vi "laneleftright2.vi"() -> (2 "Coeff right":dbl[](array[numeric]), 3 "Coeff left":dbl[](array[numeric]))   [LabVIEW 2015]
uses:
  G_SEN.vi
  <vilib>/Analysis/1siggen.llb/Ramp Pattern by Delta.vi
  G_LCM.vi
  <vilib>/Analysis/polynomials.llb/1D Polynomial Evaluation (DBL).vi
  <vilib>/Analysis/NI_AALPro.lvlib
  <vilib>/Analysis/NI_AALBase.lvlib
panel:
  in  "poly":i32=5
  out "Coeff stop":dbl[](array[numeric])
  out "y_mobileye":dbl[](array[numeric])=[0.8601491478953653, 0.8717844136967624, 0.882947592858927, 0.8936326403234123, 0.9038337699485205, 0.9135454576426009, 0.9227624443554423, 0.9314797389261423, 0.9396926207859084, 0.9473966425143293, 0.9545876322477319, 0.9612616959383189, 0.9674152194628639, 0.9730448705798238, 0.9781476007338057, 0.9827206467064133, 0.9867615321125792, 0.9902680687415704, 0.993238357741943, 0.9956707906498045, 0.9975640502598242, 0.9989171113385246, 0.9997292411794617, 1.0, 0.9997292411794617, 0.9989171113385246, 0.9975640502598242, 0.9956707906498045, 0.993238357741943, 0.9902680687415704, 0.9867615321125792, 0.9827206467064133]
  in  "iter":i32=5
  out "Waveform Graph":dbl[](graph)
  out "w all":dbl[](array[numeric])
  out "c_tmp":dbl[](array[numeric])
  out "y seed":dbl[](array[numeric])
  out "XY Graph 4":cluster{"Y":dbl[], "Y":dbl[]}[](graph)=[{"Y"=array[3210 elements], "Y"=array[3210 elements]}, {"Y"=[-0.0, 0.001154394197769193, 0.004617650635850623, 0.010389990872226917, 0.018471784248973222, 0.02886354801042046, 0.041565947468740205, 0.056579796217107514, 0.0739060563904701, 0.0935458389742223, 0.11550040416098284, 0.13977116175580306, 0.16635967162997645, 0.19526764422393228, 0.2264969410994837, 0.26004957554195585, 0.2959277132125635, 0.3341336728515216, 0.374669927032528, 0.417539102969144, 0.4627439833735707, 0.5102875073687159, 0.560172771454063, 0.6124030305261954, 0.6669816989546717, 0.7239123517142048, 0.7831987255740245, 0.8448447203451934, 0.9088544001870815, 0.975231994973953, 1.0439819017227023, 1.1151086860829622, 1.1886170838907617, 1.2645120027869723, 1.342798523901962, 1.42348190360768, 1.5065675753387922, 1.592061151484188, 1.6799684253507792, 1.770295373200753, 1.8630481563645134, 1.9582331234307588, 2.0558568125157564, 2.1559259536137603, 2.258447471030621], "Y"=[0.0, 0.5, 1.0, 1.5, 2.0, 2.5, 3.0, 3.5, 4.0, 4.5, 5.0, 5.5, 6.0, 6.5, 7.0, 7.5, 8.0, 8.5, 9.0, 9.5, 10.0, 10.5, 11.0, 11.5, 12.0, 12.5, 13.0, 13.5, 14.0, 14.5, 15.0, 15.5, 16.0, 16.5, 17.0, 17.5, 18.0, 18.5, 19.0, 19.5, 20.0, 20.5, 21.0, 21.5, 22.0]}, {"Y"=[0.362252581831572], "Y"=[-0.8199241909738847]}, {"Y"=array[210 elements], "Y"=array[210 elements]}, {"Y"=[-0.925, -0.925, -0.925, -0.6775, -0.6775, -0.925, -0.925, -0.925, -0.925, -0.6775, -0.6775, -0.925, -0.925, -0.925, 0.9025, 0.9025, 0.9025, 0.6775, 0.6775, 0.9025, 0.9025, 0.9025, 0.9025, 0.6775, 0.6775, 0.9025, 0.9025, 0.9025, -0.925], "Y"=[-0.75, -0.224, 0.224, 0.224, -0.224, -0.224, 0.224, 2.415, 2.885, 2.885, 2.415, 2.415, 2.885, 3.5, 3.5, 2.885, 2.415, 2.415, 2.885, 2.885, 2.415, 0.224, -0.224, -0.224, 0.224, 0.224, -0.224, -0.75, -0.75]}, {"Y"=[0.171875, 0.15377271904051304, 0.1346290179491043, 0.11445423440635205, 0.09325870609283447, 0.07105277068912982, 0.04784676587581635, 0.02365102933347224, -0.0015241012573242174, -0.02766828821599482, -0.05477119386196136, -0.08282248051464558, -0.11181181049346922, -0.14172884611785413, -0.17256324970722198, -0.20430468358099463, -0.23694281005859374, -0.27046729145944115, -0.30486779010295867, -0.340133968308568, -0.3762554883956909, -0.41322201268374914, -0.4510232034921646, -0.4896487231403589], "Y"=[0.0, 0.5, 1.0, 1.5, 2.0, 2.5, 3.0, 3.5, 4.0, 4.5, 5.0, 5.5, 6.0, 6.5, 7.0, 7.5, 8.0, 8.5, 9.0, 9.5, 10.0, 10.5, 11.0, 11.5]}, {"Y"=[1.796875, 1.778772719040513, 1.7596290179491043, 1.739454234406352, 1.7182587060928345, 1.6960527706891297, 1.6728467658758164, 1.6486510293334722, 1.6234758987426758, 1.5973317117840051, 1.5702288061380387, 1.5421775194853544, 1.513188189506531, 1.483271153882146, 1.452436750292778, 1.4206953164190055, 1.3880571899414063, 1.354532708540559, 1.3201322098970414, 1.284866031691432, 1.248744511604309, 1.2117779873162509, 1.1739767965078354, 1.135351276859641, 1.0959117660522462, 1.0556686017662287, 1.014632121682167, 0.9728126634806396, 0.9302205648422242, 0.8868661634474992], "Y"=[0.0, 0.5, 1.0, 1.5, 2.0, 2.5, 3.0, 3.5, 4.0, 4.5, 5.0, 5.5, 6.0, 6.5, 7.0, 7.5, 8.0, 8.5, 9.0, 9.5, 10.0, 10.5, 11.0, 11.5, 12.0, 12.5, 13.0, 13.5, 14.0, 14.5]}, {"Y"=[-1.453125, -1.471227280959487, -1.4903709820508957, -1.510545765593648, -1.5317412939071655, -1.5539472293108703, -1.5771532341241836, -1.6013489706665278, -1.6265241012573242, -1.6526682882159949, -1.6797711938619613, -1.7078224805146456, -1.736811810493469, -1.766728846117854, -1.797563249707222, -1.8293046835809945, -1.8619428100585937, -1.895467291459441, -1.9298677901029586], "Y"=[0.0, 0.5, 1.0, 1.5, 2.0, 2.5, 3.0, 3.5, 4.0, 4.5, 5.0, 5.5, 6.0, 6.5, 7.0, 7.5, 8.0, 8.5, 9.0]}, {"Y"=[0.171875, 0.2568230007600336, 0.3384052130063493, 0.44574342526006827, 0.5205081969556753, 0.5917680690742042, 0.659409530134929, 0.7229937549325056, 0.7835496148685115, 0.8405449546633443, 0.9258576868463875], "Y"=[-20.239964538708662, -19.725637940364884, -19.211158961966362, -18.6998967366845, -18.19022720070031, -17.681887266143153, -17.17615515566314, -16.67683575591291, -16.176265245349786, -15.679082775270938, -15.183754484614711]}, {"Y"=[7.134647485270904], "Y"=[38.71960961082238]}, {"Y"=array[980 elements], "Y"=array[980 elements]}, {"Y"=[], "Y"=[]}]
  out "y all":dbl[](array[numeric])
  out "x all":dbl[](array[numeric])
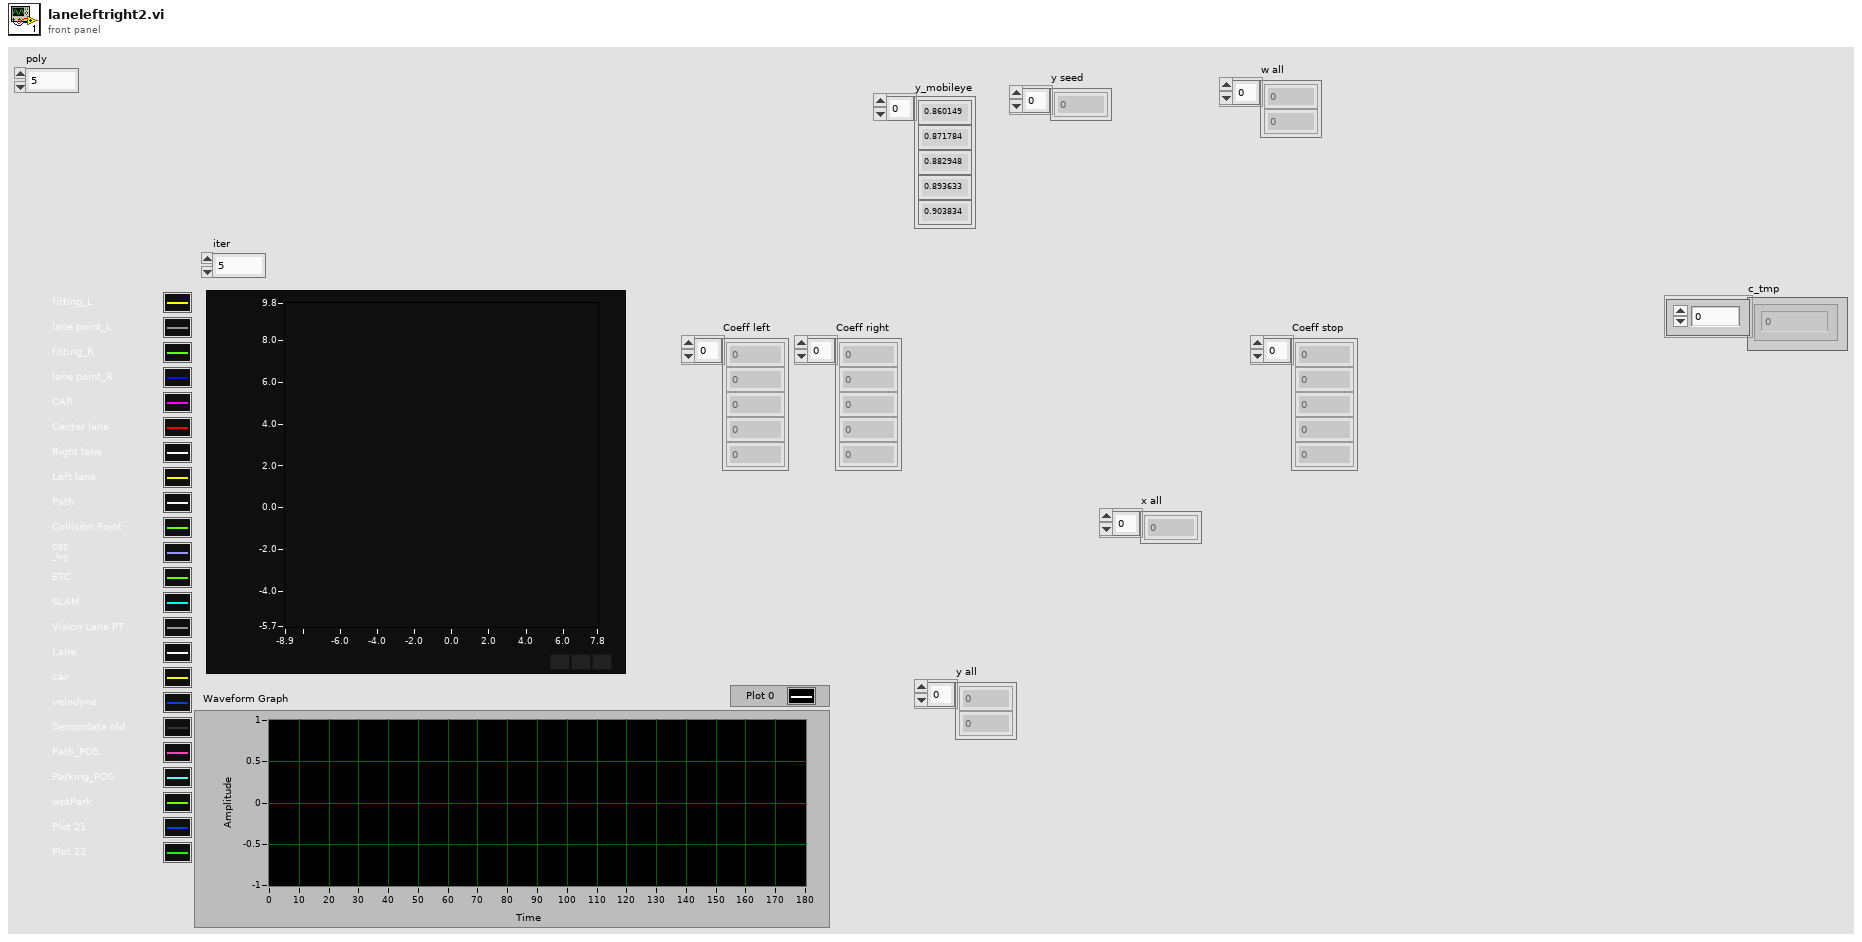
[diagram p1: front panel]
types:
  T1 = cluster{"hash":i64, "sys time":i64, "size":i64, "x":dbl[], "y":dbl[]}
  T2 = cluster{"delta":bool, "Rotational position":dbl, "Rotational position":dbl}[]
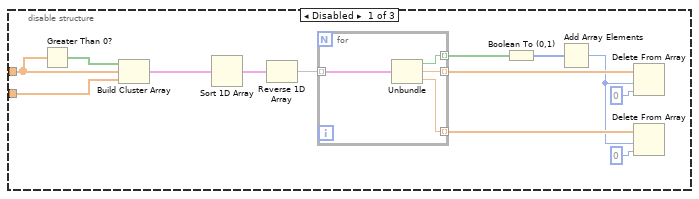
[diagram p4: hidden frame]
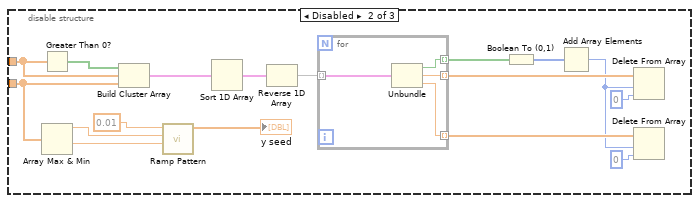
[diagram p5: hidden frame]
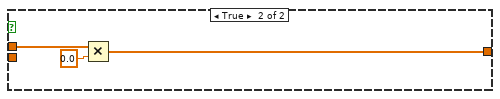
[diagram p6: hidden frame]
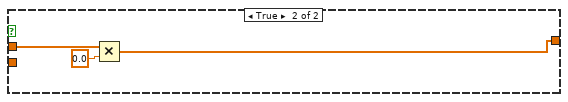
[diagram p7: hidden frame]
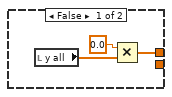
[diagram p8: hidden frame]
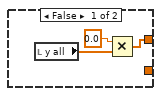
[diagram p9: hidden frame]
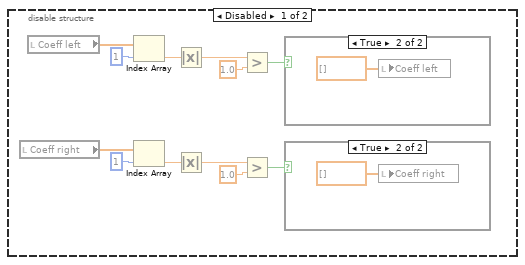
[diagram p11: hidden frame]
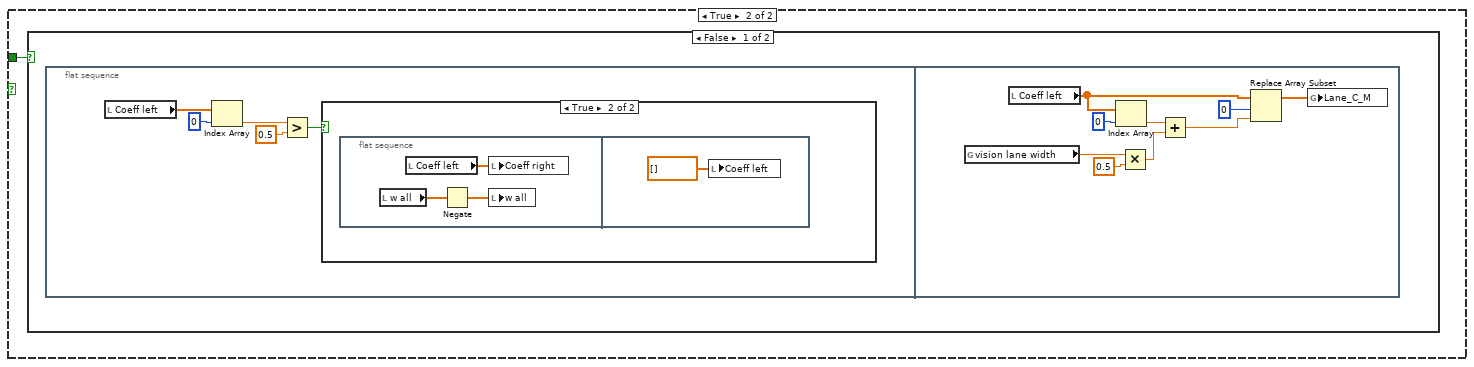
[diagram p15: hidden frame]
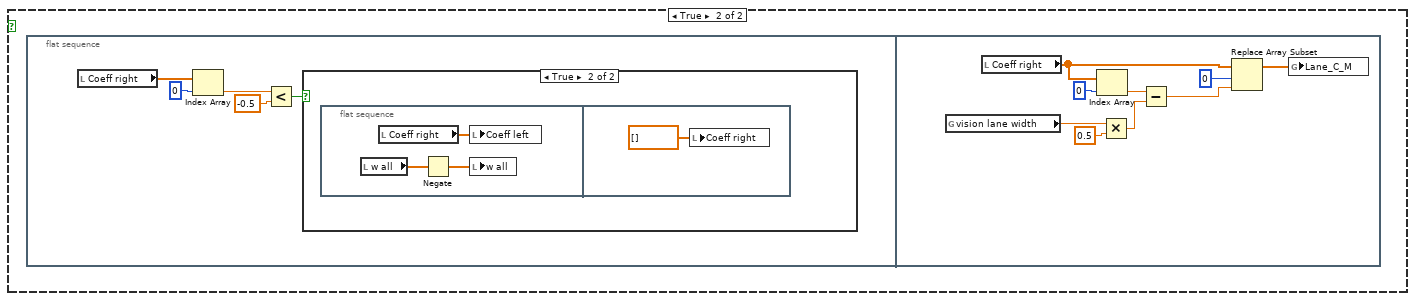
[diagram p17: hidden frame]
diagram:
  n1 = flat-sequence {
    frame #0 {
      n2 = First Call?() -> (First Call?: T/F=w1:bool)
      n3 = case shown="True" w1 {
        frame False {
        }
        frame True {
          w2 = dbl[][] [] ("Lane_R_V")
          n4 = disable-structure shown="Enabled" {
            frame Enabled {
              w8 = dbl[] [] ("Coeff left")
              n5 = local write "Coeff left"(w8) -> ()
              n6 = local write "Coeff right"(w8) -> ()
            }
            frame Disabled {
            }
          }
          n7 = global write "G_SEN.vi" "vision lane width"(3.5 ("vision lane width")) -> ()
          n8 = global write "G_SEN.vi" "Lane_L_V"(w2) -> ()
          n9 = global write "G_SEN.vi" "Lane_R_V"(w2) -> ()
          n10 = call-poly <vilib>:"Ramp Pattern.vi"("start"=-4.0, "end"=6.0, "delta"=0.1) -> ("Ramp Pattern"=→"y_mobileye":dbl[])  [unwired: 6 in, 2 out]
        }
      }
    }
    frame #1 {
      n11 = global read "G_LCM.vi" "VISION_LANE_PT"() -> (w26:T1)
      n12 = Unbundle By Name(w26) -> ("x"=w15:dbl[], "y"=w14:dbl[])
      n13 = In Range and Coerce(upper limit=6.0 ("delta"), x=w14, lower limit=-4.0) -> (In Range?=w17:bool[])  [unwired: 1 out]
      n14 = Build Cluster Array(w17, w15, w14) -> (w19:T2)
      n15 = Sort 1D Array(array=w19) -> (sorted array=w18:T2)
      n16 = Reverse 1D Array(array=w18) -> (reversed array=w24:T2)
      n17 = for {
        tunnel: w24 -> [w30] mode=indexing
        tunnel: [w29] -> w22 mode=indexing
        tunnel: [w28] -> w21 mode=indexing
        tunnel: [w27] -> w13 mode=indexing
        n18 = Unbundle(w30) -> ("delta"=w27:bool, "Rotational position"=w29:dbl, "Rotational position"=w28:dbl)
      }
      n19 = Boolean To (0,1)(Boolean=w13) -> (0, 1=w23:i16[])
      n20 = Add Array Elements(numeric array=w23) -> (sum=w12:i16)
      n21 = Delete From Array(array=w22, length=w12, index=0) -> (deleted portion=→"x all":dbl[])  [unwired: 1 out]
      n22 = Delete From Array(array=w21, length=w12, index=0) -> (deleted portion=→"y all":dbl[])  [unwired: 1 out]
    }
    frame #2 {
      n23 = local read "x all"() -> (w33:dbl[])
      n24 = local read "y all"() -> (w32:dbl[])
      n25 = disable-structure shown="Enabled" {
        disable-tunnel: w33 -> [w35 w56 w92]
        disable-tunnel: w32 -> [w46 w55 w97]
        disable-tunnel: [_ _ w72] -> w31
        frame Disabled {
          n26 = Greater Than 0?(x=w35) -> (x > 0?=w34:bool[])
          n27 = Build Cluster Array(w34, w35, w46) -> (w45:cluster{bool, dbl, dbl}[])
          n28 = Sort 1D Array(array=w45) -> (sorted array=w44:cluster{bool, dbl, dbl}[])
          n29 = Reverse 1D Array(array=w44) -> (reversed array=w43:cluster{bool, dbl, dbl}[])
          n30 = for {
            tunnel: w43 -> [w50] mode=indexing
            tunnel: [w49] -> w40 mode=indexing
            tunnel: [w48] -> w39 mode=indexing
            tunnel: [w47] -> w42 mode=indexing
            n31 = Unbundle(w50) -> (w47:bool, w49:dbl, w48:dbl)
          }
          n32 = Boolean To (0,1)(Boolean=w42) -> (0, 1=w41:i16[])
          n33 = Add Array Elements(numeric array=w41) -> (sum=w38:i16)
          n34 = Delete From Array(array=w40, length=w38, index=0) -> ()  [unwired: 2 out]
          n35 = Delete From Array(array=w39, length=w38, index=0) -> ()  [unwired: 2 out]
        }
        frame Disabled {
          n36 = Greater Than 0?(x=w56) -> (x > 0?=w57:bool[])
          n37 = Array Max & Min(array=w55) -> (max value=w54:dbl, min value=w53:dbl)  [unwired: 2 out]
          n38 = Build Cluster Array(w57, w56, w55) -> (w67:cluster{bool, dbl, dbl}[])
          n39 = call-poly <vilib>:"Ramp Pattern.vi"("start"=w53, "end"=w54, "delta"=0.01) -> ("Ramp Pattern"=→"y seed":dbl[])  [unwired: 6 in, 2 out]
          n40 = Sort 1D Array(array=w67) -> (sorted array=w66:cluster{bool, dbl, dbl}[])
          n41 = Reverse 1D Array(array=w66) -> (reversed array=w65:cluster{bool, dbl, dbl}[])
          n42 = for {
            tunnel: w65 -> [w71] mode=indexing
            tunnel: [w70] -> w62 mode=indexing
            tunnel: [w69] -> w61 mode=indexing
            tunnel: [w68] -> w64 mode=indexing
            n43 = Unbundle(w71) -> (w68:bool, w70:dbl, w69:dbl)
          }
          n44 = Boolean To (0,1)(Boolean=w64) -> (0, 1=w63:i16[])
          n45 = Add Array Elements(numeric array=w63) -> (sum=w60:i16)
          n46 = Delete From Array(array=w62, length=w60, index=0) -> ()  [unwired: 2 out]
          n47 = Delete From Array(array=w61, length=w60, index=0) -> ()  [unwired: 2 out]
        }
        frame Enabled {
          n48 = Subtract(x=w92, y=6.0) -> (x-y=w105:dbl[])
          n49 = Subtract(x=w97, y=0.0) -> (x-y=w95:dbl[])
          n50 = Subtract(x=w92, y=-6.0) -> (x-y=w103:dbl[])
          n51 = local read "Coeff left"() -> (w76:dbl[])
          n52 = Square(x=w103) -> (x^2=w104:dbl[])
          n53 = Square(x=w105) -> (x^2=w94:dbl[])
          n54 = Square(x=w95) -> (x^2=w93:dbl[])
          n55 = local read "Coeff right"() -> (w77:dbl[])
          n56 = Add(x=w104, y=w93) -> (x+y=w86:dbl[])
          n57 = Add(x=w93, y=w94) -> (x+y=w91:dbl[])
          n58 = Empty Array?(array=w76) -> (empty?=w75:bool)
          n59 = local read "y all"() -> (w79:dbl[])
          n60 = Empty Array?(array=w77) -> (empty?=w74:bool)
          n61 = In Range and Coerce(upper limit=36.0, x=w86, lower limit=4.0) -> (In Range?=w84:bool[])  [unwired: 1 out]
          n62 = In Range and Coerce(upper limit=36.0, x=w91, lower limit=4.0) -> (In Range?=w85:bool[])  [unwired: 1 out]
          n63 = local read "y all"() -> (w73:dbl[])
          n64 = case shown="False" w75 {
            tunnel: w79 -> [w126 w134]
            tunnel: w76 -> [w123 _]
            tunnel: [w121 w133] -> w78
            frame False {
              n65 = call-poly <vilib>:"Polynomial Evaluation.vi"("P(x)"=w123, "A"=w126) -> ("P(A)"=w125:dbl[])  [unwired: 1 out]
              n66 = local read "x all"() -> (w124:dbl[])
              n67 = Subtract(x=w125, y=w124) -> (x-y=w130:dbl[])
              n68 = Absolute Value(x=w130) -> (abs(x)=w129:dbl[])
              n69 = Negate(x=w129) -> (-x=w128:dbl[])
              n70 = Add(x=w128, y=1.0) -> (x+y=w132:dbl[])
              n71 = Max & Min(x=0.0, y=w132) -> (max(x,y)=w122:dbl[])  [unwired: 1 out]
              n72 = Negate(x=w122) -> (-x=w121:dbl[])
            }
            frame True {
              n73 = Multiply(x=w134, y=0.0) -> (x*y=w133:dbl[])
            }
          }
          n74 = case shown="False" w74 {
            tunnel: [w115 w118] -> w81
            tunnel: w77 -> [w114 _]
            tunnel: w73 -> [w107 w119]
            frame False {
              n75 = call-poly <vilib>:"Polynomial Evaluation.vi"("P(x)"=w114, "A"=w107) -> ("P(A)"=w112:dbl[])  [unwired: 1 out]
              n76 = local read "x all"() -> (w113:dbl[])
              n77 = Subtract(x=w112, y=w113) -> (x-y=w108:dbl[])
              n78 = Absolute Value(x=w108) -> (abs(x)=w109:dbl[])
              n79 = Negate(x=w109) -> (-x=w110:dbl[])
              n80 = Add(x=w110, y=1.0) -> (x+y=w116:dbl[])
              n81 = Max & Min(x=0.0, y=w116) -> (max(x,y)=w115:dbl[])  [unwired: 1 out]
            }
            frame True {
              n82 = Multiply(x=w119, y=0.0) -> (x*y=w118:dbl[])
            }
          }
          n83 = Boolean To (0,1)(Boolean=w84) -> (0, 1=w83:i16[])
          n84 = Boolean To (0,1)(Boolean=w85) -> (0, 1=w82:i16[])
          n85 = Multiply(x=i16 -1, y=w83) -> (x*y=w100:i16[])
          n86 = Add(x=w100, y=w82) -> (x+y=w98:i16[])
          n87 = Multiply(x=w98, y=1.0 ("element")) -> (x*y=w80:dbl[])
          n88 = Compound Arithmetic op=ADD(w80, w81, w78) -> (w72:dbl[])
        }
      }
      "w all" <- w31
    }
    frame #3 {
      n89 = for {
        N: "iter" -> [_]
        tunnel: "poly" -> [w139]
        n90 = flat-sequence {
          tunnel: [w153] -> w145
          tunnel: w139 -> [w146]
          tunnel: [w146] -> w138
          tunnel: [w184] -> w144
          tunnel: w145 -> [w184]
          tunnel: [w181] -> w142
          tunnel: w138 -> [w174]
          tunnel: w144 -> [w246]
          tunnel: [w246] -> w143
          tunnel: w142 -> [w245]
          tunnel: [w245] -> w141
          tunnel: [w216] -> w140
          tunnel: w143 -> [w254]
          tunnel: w141 -> [w253]
          tunnel: w140 -> [w252]
          frame #0 {
            n91 = local read "w all"() -> (w155:dbl[])
            n92 = Greater?(x=w155, y=0.99) -> (0:w147:bool[])
            n93 = Boolean To (0,1)(Boolean=w147) -> (0, 1=w148:i16[])
            n94 = Add Array Elements(numeric array=w148) -> (sum=w151:i16)
            n95 = Greater?(x=w151, y=i16 50) -> (0:w149:bool)
            n96 = case shown="True" w149 {
              tunnel: [w157 w164] -> w153
              tunnel: [_ w163] -> w152
              tunnel: w148 -> [_ w160]
              tunnel: w146 -> [_ w159]
              frame False {
                n97 = local read "y all"() -> (w158:dbl[])
                n98 = Multiply(x=0.0, y=w158) -> (x*y=w157:dbl[])
              }
              frame True {
                n99 = local read "x all"() -> (w161:dbl[])
                n100 = local read "y all"() -> (w162:dbl[])
                n101 = call <vilib>:"General Polynomial Fit Coefficients.vi"("Y"=w161, "polynomial order"=w159, "X"=w162, "Weight"=w160) -> ("Polynomial Coefficients"=w163:dbl[])  [unwired: 10 in, 1 out]
                n102 = local read "y all"() -> (w173:dbl[])
                n103 = call-poly <vilib>:"Polynomial Evaluation.vi"("P(x)"=w163, "A"=w173) -> ("P(A)"=w172:dbl[])  [unwired: 1 out]
                n104 = local read "x all"() -> (w171:dbl[])
                n105 = Subtract(x=w172, y=w171) -> (x-y=w170:dbl[])
                n106 = Absolute Value(x=w170) -> (abs(x)=w169:dbl[])
                n107 = Negate(x=w169) -> (-x=w168:dbl[])
                n108 = Add(x=w168, y=1.0) -> (x+y=w165:dbl[])
                n109 = Max & Min(x=0.0, y=w165) -> (max(x,y)=w164:dbl[])  [unwired: 1 out]
              }
            }
            "Coeff right" <- w152
          }
          frame #1 {
            n110 = local read "w all"() -> (w182:dbl[])
            n111 = Less?(x=w182, y=-0.99) -> (x < y?=w177:bool[])
            n112 = Boolean To (0,1)(Boolean=w177) -> (0, 1=w175:i16[])
            n113 = Add Array Elements(numeric array=w175) -> (sum=w178:i16)
            n114 = Greater?(x=w178, y=i16 50) -> (0:w176:bool)
            n115 = case shown="True" w176 {
              tunnel: [w185 w193] -> w181
              tunnel: [_ w192] -> w180
              tunnel: w175 -> [_ w189]
              tunnel: w174 -> [_ w188]
              frame False {
                n116 = local read "y all"() -> (w186:dbl[])
                n117 = Multiply(x=0.0, y=w186) -> (x*y=w185:dbl[])
              }
              frame True {
                n118 = local read "x all"() -> (w190:dbl[])
                n119 = local read "y all"() -> (w191:dbl[])
                n120 = call <vilib>:"General Polynomial Fit Coefficients.vi"("Y"=w190, "polynomial order"=w188, "X"=w191, "Weight"=w189) -> ("Polynomial Coefficients"=w192:dbl[])  [unwired: 10 in, 1 out]
                n121 = local read "y all"() -> (w197:dbl[])
                n122 = call-poly <vilib>:"Polynomial Evaluation.vi"("P(x)"=w192, "A"=w197) -> ("P(A)"=w198:dbl[])  [unwired: 1 out]
                n123 = local read "x all"() -> (w199:dbl[])
                n124 = Subtract(x=w198, y=w199) -> (x-y=w200:dbl[])
                n125 = Absolute Value(x=w200) -> (abs(x)=w201:dbl[])
                n126 = Negate(x=w201) -> (-x=w195:dbl[])
                n127 = Add(x=w195, y=1.0) -> (x+y=w202:dbl[])
                n128 = Max & Min(x=0.0, y=w202) -> (max(x,y)=w196:dbl[])  [unwired: 1 out]
                n129 = Negate(x=w196) -> (-x=w193:dbl[])
              }
            }
            "Coeff left" <- w180
          }
          frame #2 {
            n130 = local read "w all"() -> (w224:dbl[])
            n131 = local read "y all"() -> (w228:dbl[])
            n132 = Absolute Value(x=w224) -> (abs(x)=w223:dbl[])
            n133 = Greater?(x=w228, y=2.0) -> (0:w226:bool[])
            n134 = Less?(x=w223, y=0.25) -> (x < y?=w222:bool[])
            n135 = And(x=w226, y=w222) -> (x .and. y?=w225:bool[])
            n136 = Boolean To (0,1)(Boolean=w225) -> (0, 1=w244:i16[])
            n137 = local read "y all"() -> (w238:dbl[])
            n138 = local read "x all"() -> (w237:dbl[])
            n139 = call <vilib>:"General Polynomial Fit Coefficients.vi"("Y"=w238, "polynomial order"=1, "X"=w237, "Weight"=w244) -> ("Polynomial Coefficients"=w209:dbl[])  [unwired: 10 in, 1 out]
            n140 = local read "x all"() -> (w242:dbl[])
            n141 = Equal To 0?(x=w209) -> (x = 0?=w208:bool[])
            n142 = Index Array(array=w209, index=1) -> (element=w219:dbl)
            n143 = And Array Elements(Boolean array=w208) -> (logical AND=w205:bool)
            n144 = call-poly <vilib>:"Polynomial Evaluation.vi"("P(x)"=w209, "A"=w242) -> ("P(A)"=w241:dbl[])  [unwired: 1 out]
            n145 = In Range and Coerce(upper limit=0.5, x=w219, lower limit=-0.5) -> (In Range?=w207:bool)  [unwired: 1 out]
            n146 = local read "y all"() -> (w240:dbl[])
            n147 = Not(x=w205) -> (.not. x?=w204:bool)
            n148 = Subtract(x=w241, y=w240) -> (x-y=w239:dbl[])
            n149 = disable-structure shown="Enabled" {
              disable-tunnel: w207 -> [w249 _]
              disable-tunnel: [w248 _] -> w206
              disable-tunnel: w204 -> [w247 _]
              frame Enabled {
                n150 = And(x=w247, y=w249) -> (x .and. y?=w248:bool)
              }
              frame Disabled {
              }
            }
            n151 = Absolute Value(x=w239) -> (abs(x)=w236:dbl[])
            n152 = Greater?(x=w236, y=0.25 ("Numeric 2")) -> (0:w234:bool[])
            n153 = Not(x=w234) -> (.not. x?=w233:bool[])
            n154 = Boolean To (0,1)(Boolean=w234) -> (0, 1=w229:i16[])
            n155 = Boolean To (0,1)(Boolean=w233) -> (0, 1=w232:i16[])
            n156 = Select(t=w209, s=w206, f=dbl[] []) -> (s? t:f=→"Coeff stop":dbl[])
            n157 = Multiply(x=w232, y=0.5) -> (x*y=w230:dbl[])
            n158 = Add(x=w229, y=w230) -> (x+y=w215:dbl[])
            n159 = Multiply(x=w215, y=0.0) -> (x*y=w213:dbl[])
            n160 = Increment(x=w213) -> (x+1=w212:dbl[])
            n161 = Select(t=w215, s=w206, f=w212) -> (s? t:f=w216:dbl[])
          }
          frame #3 {
            n162 = local read "w all"() -> (w258:dbl[])
            n163 = Compound Arithmetic op=ADD(w258, w254, w253) -> (w251:dbl[])
            n164 = Multiply(x=w252, y=w251) -> (x*y=w250:dbl[])
            n165 = In Range and Coerce(upper limit=1.0, x=w250, lower limit=-1.0) -> (coerced(x)=w255:dbl[])  [unwired: 1 out]
            n166 = local write "w all"(w255) -> ()
          }
        }
      }
    }
    frame #4 {
      n167 = disable-structure shown="Enabled" {
        frame Disabled {
          n168 = local read "Coeff right"() -> (w261:dbl[])
          n169 = local read "Coeff left"() -> (w268:dbl[])
          n170 = Index Array(array=w268, index=1) -> (element=w267:dbl)
          n171 = Index Array(array=w261, index=1) -> (element=w262:dbl)
          n172 = Absolute Value(x=w267) -> (abs(x)=w270:dbl)
          n173 = Absolute Value(x=w262) -> (abs(x)=w259:dbl)
          n174 = Greater?(x=w270, y=1.0) -> (0:w265:bool)
          n175 = Greater?(x=w259, y=1.0) -> (0:w264:bool)
          n176 = case shown="True" w265 {
            frame False {
            }
            frame True {
              n177 = local write "Coeff left"(dbl[] [] ("Coeff left")) -> ()
            }
          }
          n178 = case shown="True" w264 {
            frame False {
            }
            frame True {
              n179 = local write "Coeff right"(dbl[] [] ("Coeff left")) -> ()
            }
          }
        }
        frame Enabled {
          w289 = 4 ("Numeric 2")
          n180 = local read "Coeff right"() -> (w291:dbl[])
          n181 = local read "Coeff left"() -> (w293:dbl[])
          n182 = Array Subset(array=w293, index=0, length=w289) -> (w274:dbl[])
          n183 = Array Subset(array=w291, index=0, length=w289) -> (w283:dbl[])
          n184 = Index Array(array=w274, index=1) -> (element=w276:dbl)
          n185 = Index Array(array=w283, index=1) -> (element=w287:dbl)
          n186 = Absolute Value(x=w276) -> (abs(x)=w277:dbl)
          n187 = Absolute Value(x=w287) -> (abs(x)=w286:dbl)
          n188 = Less?(x=w277, y=1.0) -> (x < y?=w279:bool)
          n189 = Less?(x=w286, y=1.0) -> (x < y?=w284:bool)
          n190 = Select(t=w274, s=w279, f=dbl[] []) -> (s? t:f=w273:dbl[])
          n191 = Select(t=w283, s=w284, f=dbl[] []) -> (s? t:f=w282:dbl[])
          n192 = local write "Coeff left"(w273) -> ()
          n193 = local write "Coeff right"(w282) -> ()
        }
      }
    }
    frame #5 {
      n194 = disable-structure shown="Enabled" {
        frame Enabled {
          n195 = local read "Coeff right"() -> (w297:dbl[])
          n196 = local read "Coeff left"() -> (w298:dbl[])
          n197 = Empty Array?(array=w298) -> (empty?=w294:bool)
          n198 = Empty Array?(array=w297) -> (empty?=w296:bool)
          n199 = Exclusive Or(1:w296, 2:w294) -> (0:w295:bool)
          n200 = case shown="False" w295 {
            tunnel: w294 -> [_ w320]
            frame False {
              n201 = flat-sequence {
                frame #0 {
                  n202 = local read "Coeff right"() -> (w302:dbl[])
                  n203 = local read "Coeff left"() -> (w303:dbl[])
                  n204 = Index Array(array=w303) -> (element=w301:dbl)  [unwired: 1 in]
                  n205 = Index Array(array=w302) -> (element=w300:dbl)  [unwired: 1 in]
                  n206 = Greater?(x=w301, y=w300) -> (0:w299:bool)
                  n207 = case shown="True" w299 {
                    frame False {
                    }
                    frame True {
                      n208 = flat-sequence {
                        frame #0 {
                          n209 = local read "Coeff right"() -> (→"c_tmp":dbl[])
                        }
                        frame #1 {
                          n210 = local read "w all"() -> (w306:dbl[])
                          n211 = local read "Coeff left"() -> (w307:dbl[])
                          n212 = Negate(x=w306) -> (-x=w305:dbl[])
                          n213 = local write "Coeff right"(w307) -> ()
                          n214 = local write "w all"(w305) -> ()
                        }
                        frame #2 {
                          n215 = local read "c_tmp"() -> (w308:dbl[])
                          n216 = local write "Coeff left"(w308) -> ()
                        }
                      }
                    }
                  }
                }
                frame #1 {
                  n217 = local read "Coeff right"() -> (w314:dbl[])
                  n218 = local read "Coeff left"() -> (w317:dbl[])
                  n219 = local read "Coeff left"() -> (w313:dbl[])
                  n220 = Subtract(x=w314, y=w317) -> (x-y=w316:dbl[])
                  n221 = Add(x=w313, y=w314) -> (x+y=w319:dbl[])
                  n222 = Index Array(array=w316, index=0) -> (element=w311:dbl)
                  n223 = Multiply(x=w319, y=0.5) -> (x*y=w312:dbl[])
                  n224 = global write "G_SEN.vi" "Lane_C_M"(w312) -> ()
                  n225 = Max & Min(x=w311, y=3.2) -> (max(x,y)=w310:dbl)  [unwired: 1 out]
                  n226 = global write "G_SEN.vi" "vision lane width"(w310) -> ()
                }
              }
            }
            frame True {
              n227 = case shown="False" w320 {
                frame False {
                  n228 = flat-sequence {
                    frame #0 {
                      n229 = local read "Coeff left"() -> (w325:dbl[])
                      n230 = Index Array(array=w325, index=0) -> (element=w323:dbl)
                      n231 = Greater?(x=w323, y=0.5) -> (0:w321:bool)
                      n232 = case shown="True" w321 {
                        frame False {
                        }
                        frame True {
                          n233 = flat-sequence {
                            frame #0 {
                              n234 = local read "w all"() -> (w327:dbl[])
                              n235 = local read "Coeff left"() -> (w328:dbl[])
                              n236 = Negate(x=w327) -> (-x=w326:dbl[])
                              n237 = local write "Coeff right"(w328) -> ()
                              n238 = local write "w all"(w326) -> ()
                            }
                            frame #1 {
                              n239 = local write "Coeff left"(dbl[] []) -> ()
                            }
                          }
                        }
                      }
                    }
                    frame #1 {
                      n240 = global read "G_SEN.vi" "vision lane width"() -> (w338:dbl)
                      n241 = local read "Coeff left"() -> (w336:dbl[])
                      n242 = Index Array(array=w336, index=0) -> (element=w334:dbl)
                      n243 = Multiply(x=w338, y=0.5) -> (x*y=w333:dbl)
                      n244 = Add(x=w334, y=w333) -> (x+y=w332:dbl)
                      n245 = Replace Array Subset(array=w336, new element=w332, index=0) -> (w330:dbl[])
                      n246 = global write "G_SEN.vi" "Lane_C_M"(w330) -> ()
                    }
                  }
                }
                frame True {
                  n247 = flat-sequence {
                    frame #0 {
                      n248 = local read "Coeff right"() -> (w343:dbl[])
                      n249 = Index Array(array=w343, index=0) -> (element=w341:dbl)
                      n250 = Less?(x=w341, y=-0.5) -> (x < y?=w339:bool)
                      n251 = case shown="True" w339 {
                        frame False {
                        }
                        frame True {
                          n252 = flat-sequence {
                            frame #0 {
                              n253 = local read "w all"() -> (w345:dbl[])
                              n254 = local read "Coeff right"() -> (w346:dbl[])
                              n255 = Negate(x=w345) -> (-x=w344:dbl[])
                              n256 = local write "Coeff left"(w346) -> ()
                              n257 = local write "w all"(w344) -> ()
                            }
                            frame #1 {
                              n258 = local write "Coeff right"(dbl[] []) -> ()
                            }
                          }
                        }
                      }
                    }
                    frame #1 {
                      n259 = global read "G_SEN.vi" "vision lane width"() -> (w356:dbl)
                      n260 = local read "Coeff right"() -> (w354:dbl[])
                      n261 = Index Array(array=w354, index=0) -> (element=w352:dbl)
                      n262 = Multiply(x=w356, y=0.5) -> (x*y=w351:dbl)
                      n263 = Subtract(x=w352, y=w351) -> (x-y=w350:dbl)
                      n264 = Replace Array Subset(array=w354, new element=w350, index=0) -> (w348:dbl[])
                      n265 = global write "G_SEN.vi" "Lane_C_M"(w348) -> ()
                    }
                  }
                }
              }
            }
          }
        }
        frame Disabled {
        }
      }
    }
    frame #6 {
      n266 = local read "w all"() -> (→"Waveform Graph":dbl[])
      n267 = disable-structure shown="Enabled" {
        frame Enabled {
          n268 = local read "Coeff right"() -> (w358:dbl[])
          n269 = local read "Coeff left"() -> (w359:dbl[])
          n270 = global write "G_SEN.vi" "Lane_R_M"(w358) -> ()
          n271 = global write "G_SEN.vi" "Lane_L_M"(w359) -> ()
        }
        frame Disabled {
        }
      }
    }
    frame #7 {
      n272 = local read "w all"() -> (w425:dbl[])
      n273 = local read "w all"() -> (w405:dbl[])
      n274 = Equal?(x=w405, y=1.0) -> (x = y?=w407:bool[])
      n275 = Equal?(x=w425, y=-1.0) -> (x = y?=w423:bool[])
      n276 = local read "x all"() -> (w422:dbl[])
      n277 = local read "y all"() -> (w421:dbl[])
      n278 = local read "x all"() -> (w408:dbl[])
      n279 = local read "y all"() -> (w409:dbl[])
      n280 = Build Cluster Array(w423, w422, w421) -> (w420:cluster{bool, dbl, dbl}[])
      n281 = Build Cluster Array(w407, w408, w409) -> (w410:cluster{bool, dbl, dbl}[])
      n282 = Sort 1D Array(array=w420) -> (sorted array=w419:cluster{bool, dbl, dbl}[])
      n283 = Sort 1D Array(array=w410) -> (sorted array=w411:cluster{bool, dbl, dbl}[])
      n284 = Reverse 1D Array(array=w419) -> (reversed array=w418:cluster{bool, dbl, dbl}[])
      n285 = Reverse 1D Array(array=w411) -> (reversed array=w412:cluster{bool, dbl, dbl}[])
      n286 = for {
        tunnel: w418 -> [w440] mode=indexing
        tunnel: [w438] -> w417 mode=indexing
        tunnel: [w437] -> w396 mode=indexing
        tunnel: [w436] -> w416
        i -> [w436]
        stop <- w439 continue-if-true
        n287 = Unbundle(w440) -> (w439:bool, w438:dbl, w437:dbl)
      }
      n288 = for {
        tunnel: w412 -> [w435] mode=indexing
        tunnel: [w433] -> w413 mode=indexing
        tunnel: [w432] -> w390 mode=indexing
        tunnel: [w431] -> w414
        i -> [w431]
        stop <- w434 continue-if-true
        n289 = Unbundle(w435) -> (w434:bool, w433:dbl, w432:dbl)
      }
      n290 = Array Subset(array=w417, index=0, length=w416) -> (w415:dbl[])
      n291 = Array Subset(array=w396, index=0, length=w416) -> (w389:dbl[])
      n292 = Array Subset(array=w413, index=0, length=w414) -> (w404:dbl[])
      n293 = Array Subset(array=w390, index=0, length=w414) -> (w385:dbl[])
      n294 = call "Convert to Dynamic Data4"("Array"=w415) -> ("Dynamic Data Type"=w374:dynamicdata)  [unwired: 3 in]
      n295 = Array Max & Min(array=w389) -> (max value=w400:dbl, min value=w398:dbl)  [unwired: 2 out]
      n296 = call "Convert to Dynamic Data3"("Array"=w389) -> ("Dynamic Data Type"=w386:dynamicdata)  [unwired: 3 in]
      n297 = call "Convert to Dynamic Data6"("Array"=w404) -> ("Dynamic Data Type"=w372:dynamicdata)  [unwired: 3 in]
      n298 = Array Max & Min(array=w385) -> (max value=w392:dbl, min value=w394:dbl)  [unwired: 2 out]
      n299 = call "Convert to Dynamic Data8"("Array"=w385) -> ("Dynamic Data Type"=w384:dynamicdata)  [unwired: 3 in]
      n300 = Increment(x=w400) -> (x+1=w399:dbl)
      n301 = Decrement(x=w398) -> (x-1=w397:dbl)
      n302 = Increment(x=w392) -> (x+1=w393:dbl)
      n303 = Decrement(x=w394) -> (x-1=w395:dbl)
      n304 = local read "y_mobileye"() -> (w402:dbl[])
      n305 = local read "Coeff stop"() -> (w403:dbl[])
      n306 = call-poly <vilib>:"Ramp Pattern.vi"("start"=w397, "end"=w399, "delta"=0.01) -> ("Ramp Pattern"=w361:dbl[])  [unwired: 6 in, 2 out]
      n307 = call-poly <vilib>:"Ramp Pattern.vi"("start"=w395, "end"=w393, "delta"=0.01) -> ("Ramp Pattern"=w360:dbl[])  [unwired: 6 in, 2 out]
      n308 = local read "Coeff right"() -> (w428:dbl[])
      n309 = local read "Coeff left"() -> (w429:dbl[])
      n310 = local read "y all"() -> (w427:dbl[])
      n311 = call-poly <vilib>:"Polynomial Evaluation.vi"("P(x)"=w403, "A"=w402) -> ("P(A)"=w368:dbl[])  [unwired: 1 out]
      n312 = local read "y_mobileye"() -> (w369:dbl[])
      n313 = local read "x all"() -> (w426:dbl[])
      n314 = call-poly <vilib>:"Polynomial Evaluation.vi"("P(x)"=w429, "A"=w361) -> ("P(A)"=w367:dbl[])  [unwired: 1 out]
      n315 = call-poly <vilib>:"Polynomial Evaluation.vi"("P(x)"=w428, "A"=w360) -> ("P(A)"=w362:dbl[])  [unwired: 1 out]
      n316 = call "Convert to Dynamic Data7"("Array"=w361) -> ("Dynamic Data Type"=w371:dynamicdata)  [unwired: 3 in]
      n317 = call "Convert to Dynamic Data11"("Array"=w360) -> ("Dynamic Data Type"=w370:dynamicdata)  [unwired: 3 in]
      n318 = call "Convert to Dynamic Data10"("Array"=w427) -> ("Dynamic Data Type"=w382:dynamicdata)  [unwired: 3 in]
      n319 = call "Convert to Dynamic Data"("Array"=w368) -> ("Dynamic Data Type"=w380:dynamicdata)  [unwired: 3 in]
      n320 = Build Array(w367, w361) -> (w366:dbl[][])
      n321 = call "Convert to Dynamic Data2"("Array"=w367) -> ("Dynamic Data Type"=w375:dynamicdata)  [unwired: 3 in]
      n322 = call "Convert to Dynamic Data9"("Array"=w426) -> ("Dynamic Data Type"=w383:dynamicdata)  [unwired: 3 in]
      n323 = Merge Signals(w371, w386, w370, w384, w382, w380) -> (w387:dynamicdata)
      n324 = call "Convert to Dynamic Data5"("Array"=w362) -> ("Dynamic Data Type"=w373:dynamicdata)  [unwired: 3 in]
      n325 = Build Array(w362, w360) -> (w363:dbl[][])
      n326 = call "Convert to Dynamic Data12"("Array"=w369) -> ("Dynamic Data Type"=w381:dynamicdata)  [unwired: 3 in]
      n327 = Transpose 2D Array(2D array=w366) -> (transposed array=w365:dbl[][])
      n328 = Merge Signals(w375, w374, w373, w372, w383, w381) -> (w388:dynamicdata)
      n329 = Transpose 2D Array(2D array=w363) -> (transposed array=w364:dbl[][])
      n330 = global write "G_SEN.vi" "Lane_L_V"(w365) -> ()
      n331 = call "Build XY Graph"("Y Input"=w387, "X Input"=w388) -> ("XY Graph"=→"XY Graph 4":cluster{"X":dbl[], "Y":dbl[]}[])  [unwired: 8 in, 1 out]
      n332 = global write "G_SEN.vi" "Lane_R_V"(w364) -> ()
    }
  }
